vi "CSP_addPaths.vi"(8 "error in":errorcluster, 9 "ClassId":i32, 10 "Selected Paths":path[](array[path]) caption="selected paths", 11 "CSP.lvclass in":refnum<class "CSP.lvclass">) -> (0 "error out":errorcluster, 3 "CSP.lvclass out":refnum<class "CSP.lvclass">)   [LabVIEW 2016, in "Spatial Pattern Filter.lvlib" / "CSP.lvclass"]
uses:
  CSP.lvclass
  _XML_EEG_File_Parser/_vlib/XML_EEG_File.lvclass
  CSP.lvclass/CSP.ctl
  <vilib>/xml/Load XML File.vi
  <vilib>/xml/NI_XML.lvlib
panel:
  # "This VI is a part of BCI Design library, http://www.ru-bci.org \nCopyright © 2020, Sotnikov Peter, All rights reserved. License: GNU GPLv3"
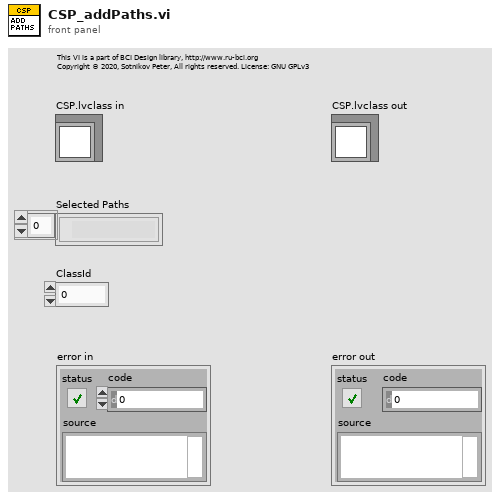
[diagram p1: front panel]
types:
  T1 = typedef "XML_EEG_File_Parser.lvlib/XML_EEG_Header.ctl" = cluster{"Attributes":cluster{"ChannelDataType":string, "NumberOfChannels":i32, "SampleRateHz":dbl, "MarkerChannel":i32}, "Body":cluster{"PatientSpecificData":string, "NumberOfDatasets":i32, "Channels":string[]}}
  T2 = typedef "XML_EEG_File_Parser.lvlib/XML_EEG_Dataset.ctl" = cluster{"Attributes":cluster{"NumberOfSamples":i32, "StartDateTime":timestamp}, "Body":cluster{"MarkerValue":string, "Channels":waveform(dbl)[]}}
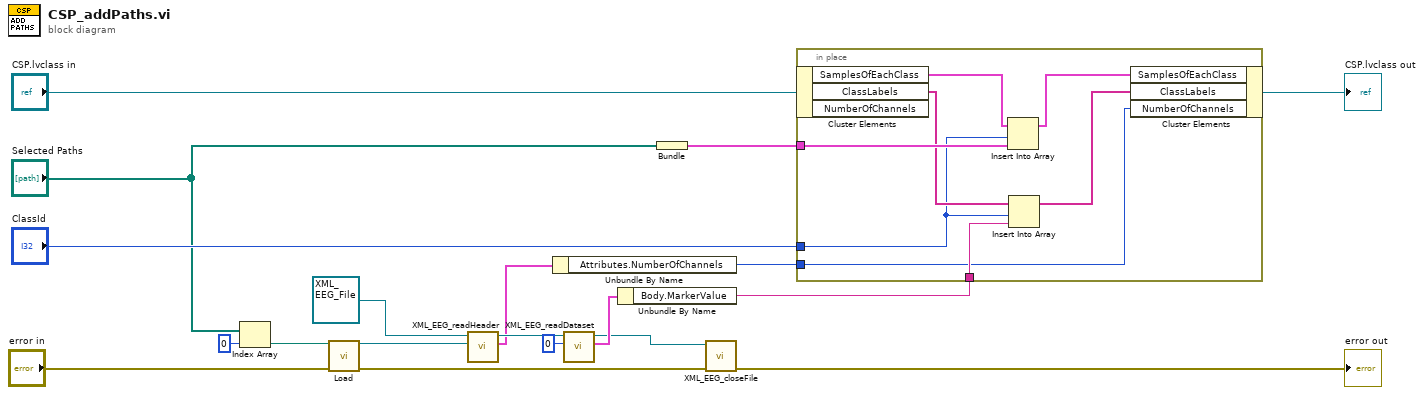
[diagram p0: block diagram]
diagram:
  n1 = Index Array(array="Selected Paths", index=0) -> (element=w15:path)
  n2 = call-poly <vilib>:"Load.vi"("path to XML document"=w15, "error in (no error)"="error in") -> ("DOM document out"=w13:refnum<k20>, "error out"=w6:errorcluster)  [unwired: 11 in, 1 out]
  n3 = call "XML_EEG_readHeader.vi"("DOM document in"=w13, "XML_EEG_Class in"=refnum<class "XML_EEG_File.lvclass"> refnum ("XML_EEG_File_Parser.lvlib:XML_EEG_File.lvclass")) -> ("XML Header out"=w4:T1, "XML_EEG_Class out"=w11:refnum<class "XML_EEG_File.lvclass">)  [unwired: 7 in, 1 out]
  n4 = Unbundle By Name(w4) -> ("Attributes.NumberOfChannels"=w3:i32)
  n5 = call "XML_EEG_readDataset.vi"("DatasetNumber"=0, "XML_EEG_File in"=w11) -> ("XML Dataset out"=w9:T2, "XML_EEG_File out"=w7:refnum<class "XML_EEG_File.lvclass">)  [unwired: 7 in, 1 out]
  n6 = Unbundle By Name(w9) -> ("Body.MarkerValue"=w8:string)
  n7 = Bundle("Selected Paths"="Selected Paths") -> (w1:cluster{"Selected Paths":path[]})  [unwired: 1 in]
  n8 = call "XML_EEG_closeFile.vi"("error in (no error)"=w6, "XML_EEG_File.lvclass"=w7) -> ("error out"=→"error out":errorcluster)  [unwired: 9 in]
  n9 = in-place {
    in-place-border: "ClassId" -> [w23]
    in-place-border: w1 -> [w26]
    in-place-border: w8 -> [w22]
    in-place-border: w3 -> [w20]
    n10 = in-place-cluster #1("CSP.lvclass in") -> ("SamplesOfEachClass"=w27:cluster{"ArrayOfFiles":path[]}[], "ClassLabels"=w24:string[])  [unwired: 1 out]
    n11 = Insert Into Array(array=w27, index=w23, new element=w26) -> (w25:cluster{"ArrayOfFiles":path[]}[])
    n12 = Insert Into Array(array=w24, index=w23, new element=w22) -> (w21:string[])
    n13 = in-place-cluster #1("SamplesOfEachClass"=w25, "ClassLabels"=w21, "NumberOfChannels"=w20) -> (→"CSP.lvclass out":refnum<class "CSP.lvclass">)
  }
